vi "CheckIfBaseTypesMatch.vi"(8 "error in (no error)":errorcluster, 10 "Actual data type":variant, 11 "Expected data type":variant) -> (0 "error out":errorcluster, 3 "types match":bool)   [LabVIEW 2015, in "VeriStandTestUtilities.lvlib"]
uses:
  VeriStandTestUtilities.lvlib
  <vilib>/Utility/Data Type/NI_Data Type.lvlib
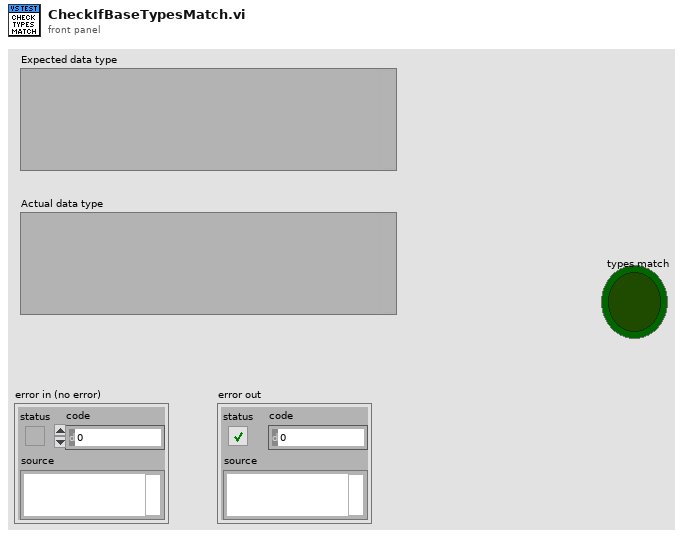
[diagram p1: front panel]
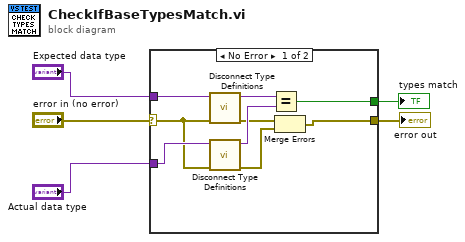
[diagram p0: block diagram]
diagram:
  n1 = case shown="No Error" "error in (no error)" {
    selector: "error in (no error)" -> [w7 w15]
    tunnel: "Expected data type" -> [w14 _]
    tunnel: "Actual data type" -> [w13 _]
    tunnel: [w8 w15] -> w3
    tunnel: [w6 _] -> w1
    frame No Error {
      n2 = call <vilib>:"Disconnect Type Definitions.vi"("error in (no error)"=w7, "Variant in"=w14) -> ("error out"=w10:errorcluster, "Variant out"=w12:variant)  [unwired: 8 in]
      n3 = call <vilib>:"Disconnect Type Definitions.vi"("error in (no error)"=w7, "Variant in"=w13) -> ("error out"=w9:errorcluster, "Variant out"=w11:variant)  [unwired: 8 in]
      n4 = Equal?(x=w12, y=w11) -> (x = y?=w6:bool)
      n5 = Merge Errors(w10, w9) -> (w8:errorcluster)
    }
    frame Error {
    }
  }
  "error out" <- w3
  "types match" <- w1
